vi "1.vi"   [LabVIEW 2015]
doc: "This VI is called when autonomous begins, and will automatically be terminated when autonomous ends. You can carry out timed or sensor driven robot movement independently without needing to return to the caller."
uses:
  <vilib>/Rock Robotics/WPI/Utilities/WPI_GetSetVariantRefNum.vi
  <vilib>/Rock Robotics/Network Tables/NT Read Number.vi
  <vilib>/Rock Robotics/WPI/RobotDrive/WPI_RobotDriveMecanumDrive_Cartesian.vi
  <vilib>/Rock Robotics/Network Tables/NT Write Numeric Array.vi
  Robot Global Data.vi
panel:
  # "Be sure to right-click and choose Data Operations>>Make Current Value default if you want to save the array values with the VI"
types:
  T1 = typedef "WPI_JoystickDevRef.ctl" = cluster{"Device":T2}
  T2 = typedef "WPI_JoystickDeviceEnum.ctl" = enum16{"USB 0", "USB 1", "USB 2", "USB 3", "USB 4", "USB 5"}
  T3 = typedef "WPI_RobotDriveDevRef.ctl" = cluster{"DevStatus":errorcluster, "Motors[]":T4[], "Square Inputs":bool, "Max Output":dbl}
  T4 = typedef "WPI_MotorControlDeviceRef.ctl" = cluster{"DeviceStatus":errorcluster, "Type":T5, "PWM":cluster{"PWM Channel":T6, "DeadBand":T7}, "CAN":cluster{"Device Number":u8, "Control Mode":T8, "Semaphore":T9, "Max Vout":dbl, "TalonSRX Control Mode":T10}, "Invert":bool}
  T5 = typedef "WPI_MotorControlType.ctl" = enum16{"PWM", "CAN", "CANTalonSRX"}
  T6 = typedef "FPGA_DIOPWMChannel.ctl" = enum8{"PWM 0", "PWM 1", "PWM 2", "PWM 3", "PWM 4", "PWM 5", "PWM 6", "PWM 7", "PWM 8", "PWM 9", "PWM MXP 0", "PWM MXP 1", "PWM MXP 2", "PWM MXP 3", "PWM MXP 4", "PWM MXP 5", "PWM MXP 6", "PWM MXP 7", "PWM MXP 8", "PWM MXP 9", "Invalid"}
  T7 = typedef "WPI_PWMDeadband.ctl" = cluster{"Name":string, "maxPositivePwm":i32, "minPositivePwm":i32, "centerPwm":i32, "maxNegativePwm":i32, "minNegativePwm":i32, "angularRange":u16}
  T8 = typedef "WPI_CANJaguar_ControlMode.ctl" = enum8{"Percent VBus", "Current", "Speed", "Position", "Voltage"}
  T9 = typedef "Semaphore RefNum" = refnum<k1>
  T10 = typedef "WPI_CANTalonSRX_APIControlMode.ctl" = enum8{"Percent VBus", "Speed", "Position", "Slave", "Unchanged / Invalid", "Voltage Compensation", "Current", "Motion Profile"}
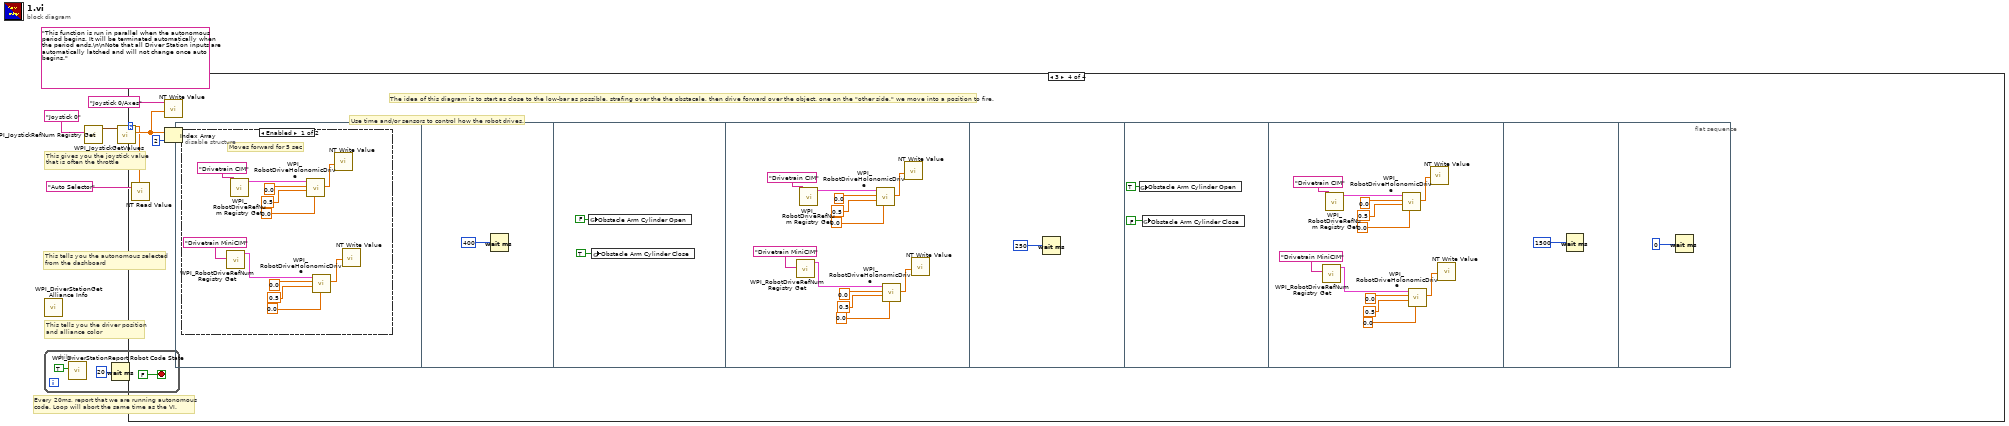
[diagram p0: block diagram]
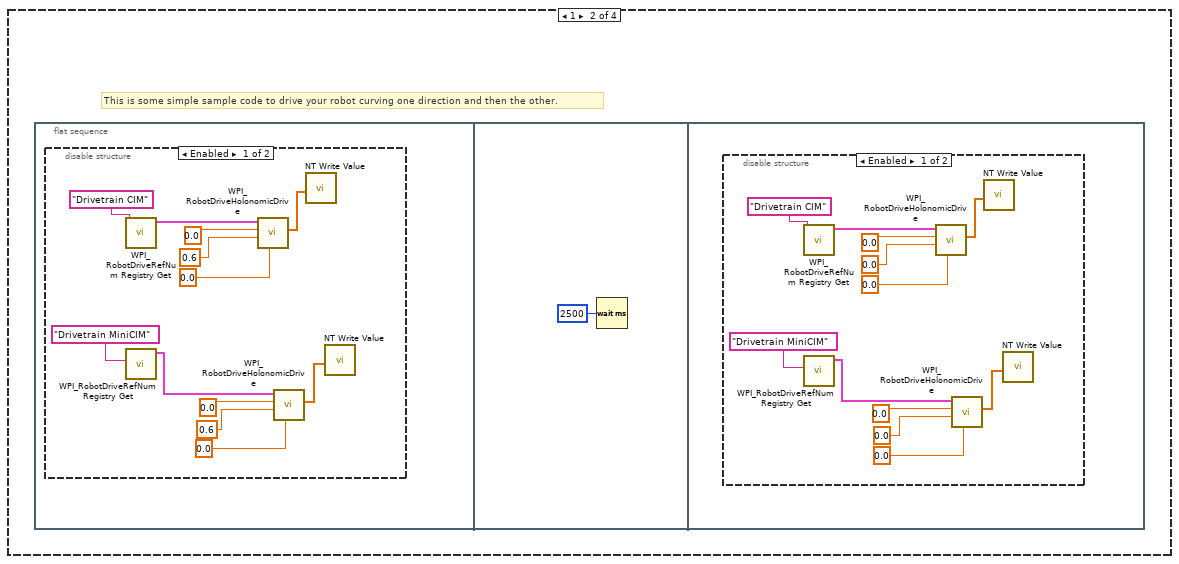
[diagram p3: hidden frame]
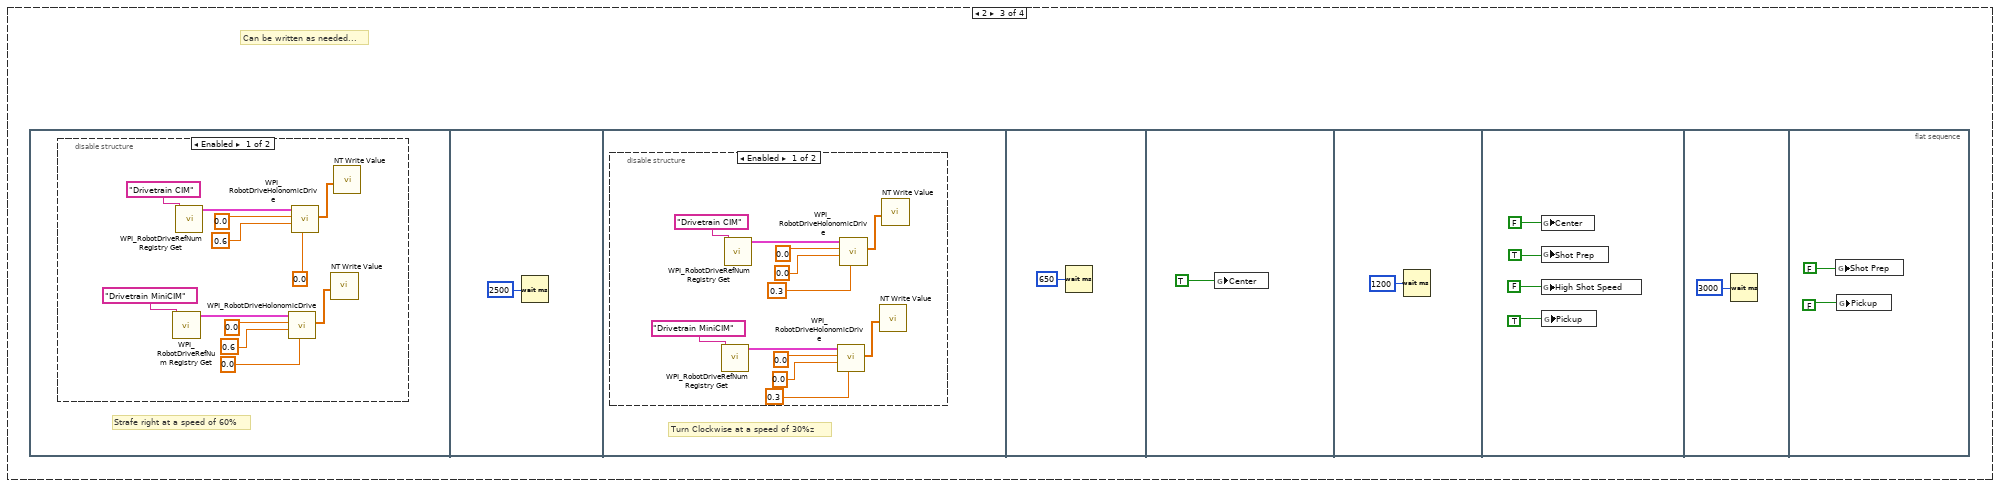
[diagram p6: hidden frame]
diagram:
  (unwired) "This function is run in parallel when the autonomous period begins. It will be terminated automatically when the period ends.\n\nNote that all Driver Station inputs are automatically latched and will not change once auto begins."
  # "This tells you the autonomous selected\nfrom the dashboard"
  # "Every 20ms, report that we are running autonomous\ncode. Loop will abort the same time as the VI."
  # "This gives you the joystick value\nthat is often the throttle"
  # "Use time and/or sensors to control how the robot drives."
  # "This tells you the driver position\nand alliance color"
  n1 = while {
    stop <- FALSE stop-if-true
    n2 = call <vilib>:"WPI_DriverStationReport Robot Code State.vi"("Autonomous"=TRUE) -> ()  [unwired: 10 in, 1 out]
    n3 = Wait (ms)(milliseconds to wait=u32 20) -> ()  [unwired: 1 out]
  }
  n4 = call <vilib>:"WPI_DriverStationGet Alliance Info.vi"() -> ()  [unwired: 12 out]
  n5 = call <vilib>:"WPI_JoystickRefNum Registry Get.vi"("refnum name"="Joystick 0") -> ("JoystickDevRef"=w6:T1)  [unwired: 1 in, 9 out]
  n6 = call <vilib>:"WPI_JoystickGetValues.vi"("JoystickDevRef"=w6) -> ("Axes"=w3:dbl[])  [unwired: 6 in, 4 out]
  n7 = call-poly <vilib>:"NT Read Value.vi"("Name"="Auto Selector") -> ("Numeric"=w1:dbl)  [unwired: 9 in, 1 out]
  n8 = case shown="3" w1 {
    frame 0, Default {
    }
    frame 1 {
      # "This is some simple sample code to drive your robot curving one direction and then the other."
      n9 = flat-sequence {
        frame #0 {
          n10 = disable-structure shown="Enabled" {
            frame Enabled {
              n11 = call <vilib>:"WPI_RobotDriveRefNum Registry Get.vi"("refnum name"="Drivetrain CIM") -> ("RobotDriveDevRef"=w18:T3)  [unwired: 1 in, 9 out]
              n12 = call <vilib>:"WPI_RobotDriveRefNum Registry Get.vi"("refnum name"="Drivetrain MiniCIM") -> ("RobotDriveDevRef"=w12:T3)  [unwired: 1 in, 9 out]
              n13 = call-poly <vilib>:"WPI_RobotDriveHolonomicDrive.vi"("Rotation"=0.0, "Y"=0.6 ("X axis value"), "X"=0.0 ("X axis value"), "RobotDriveDevRef"=w18) -> ("Motor Values"=w19:dbl[])  [unwired: 5 in, 2 out]
              n14 = call-poly <vilib>:"WPI_RobotDriveHolonomicDrive.vi"("Rotation"=0.0, "Y"=0.6 ("X axis value"), "X"=0.0 ("X axis value"), "RobotDriveDevRef"=w12) -> ("Motor Values"=w14:dbl[])  [unwired: 5 in, 2 out]
              n15 = call-poly <vilib>:"NT Write Value.vi"("Numeric Array"=w19) -> ()  [unwired: 10 in, 1 out]
              n16 = call-poly <vilib>:"NT Write Value.vi"("Numeric Array"=w14) -> ()  [unwired: 10 in, 1 out]
            }
            frame Disabled {
            }
          }
        }
        frame #1 {
          n17 = Wait (ms)(milliseconds to wait=u32 2500) -> ()  [unwired: 1 out]
        }
        frame #2 {
          n18 = disable-structure shown="Enabled" {
            frame Enabled {
              n19 = call <vilib>:"WPI_RobotDriveRefNum Registry Get.vi"("refnum name"="Drivetrain CIM") -> ("RobotDriveDevRef"=w31:T3)  [unwired: 1 in, 9 out]
              n20 = call <vilib>:"WPI_RobotDriveRefNum Registry Get.vi"("refnum name"="Drivetrain MiniCIM") -> ("RobotDriveDevRef"=w25:T3)  [unwired: 1 in, 9 out]
              n21 = call-poly <vilib>:"WPI_RobotDriveHolonomicDrive.vi"("Rotation"=0.0, "Y"=0.0 ("X axis value"), "X"=0.0 ("X axis value"), "RobotDriveDevRef"=w31) -> ("Motor Values"=w32:dbl[])  [unwired: 5 in, 2 out]
              n22 = call-poly <vilib>:"WPI_RobotDriveHolonomicDrive.vi"("Rotation"=0.0, "Y"=0.0 ("X axis value"), "X"=0.0 ("X axis value"), "RobotDriveDevRef"=w25) -> ("Motor Values"=w27:dbl[])  [unwired: 5 in, 2 out]
              n23 = call-poly <vilib>:"NT Write Value.vi"("Numeric Array"=w32) -> ()  [unwired: 10 in, 1 out]
              n24 = call-poly <vilib>:"NT Write Value.vi"("Numeric Array"=w27) -> ()  [unwired: 10 in, 1 out]
            }
            frame Disabled {
            }
          }
        }
      }
    }
    frame 2 {
      # "Can be written as needed..."
      n25 = flat-sequence {
        frame #0 {
          # "Strafe right at a speed of 60%"
          n26 = disable-structure shown="Enabled" {
            frame Enabled {
              n27 = call <vilib>:"WPI_RobotDriveRefNum Registry Get.vi"("refnum name"="Drivetrain MiniCIM") -> ("RobotDriveDevRef"=w37:T3)  [unwired: 1 in, 9 out]
              n28 = call <vilib>:"WPI_RobotDriveRefNum Registry Get.vi"("refnum name"="Drivetrain CIM") -> ("RobotDriveDevRef"=w43:T3)  [unwired: 1 in, 9 out]
              n29 = call-poly <vilib>:"WPI_RobotDriveHolonomicDrive.vi"("Rotation"=0.0, "Y"=0.6 ("X axis value"), "X"=0.0 ("X axis value"), "RobotDriveDevRef"=w37) -> ("Motor Values"=w38:dbl[])  [unwired: 5 in, 2 out]
              n30 = call-poly <vilib>:"WPI_RobotDriveHolonomicDrive.vi"("Rotation"=0.0, "Y"=0.6 ("X axis value"), "X"=0.0 ("X axis value"), "RobotDriveDevRef"=w43) -> ("Motor Values"=w44:dbl[])  [unwired: 5 in, 2 out]
              n31 = call-poly <vilib>:"NT Write Value.vi"("Numeric Array"=w38) -> ()  [unwired: 10 in, 1 out]
              n32 = call-poly <vilib>:"NT Write Value.vi"("Numeric Array"=w44) -> ()  [unwired: 10 in, 1 out]
            }
            frame Disabled {
            }
          }
        }
        frame #1 {
          n33 = Wait (ms)(milliseconds to wait=u32 2500) -> ()  [unwired: 1 out]
        }
        frame #2 {
          # "Turn Clockwise at a speed of 30%z"
          n34 = disable-structure shown="Enabled" {
            frame Enabled {
              n35 = call <vilib>:"WPI_RobotDriveRefNum Registry Get.vi"("refnum name"="Drivetrain MiniCIM") -> ("RobotDriveDevRef"=w50:T3)  [unwired: 1 in, 9 out]
              n36 = call <vilib>:"WPI_RobotDriveRefNum Registry Get.vi"("refnum name"="Drivetrain CIM") -> ("RobotDriveDevRef"=w56:T3)  [unwired: 1 in, 9 out]
              n37 = call-poly <vilib>:"WPI_RobotDriveHolonomicDrive.vi"("Rotation"=0.3, "Y"=0.0 ("X axis value"), "X"=0.0 ("X axis value"), "RobotDriveDevRef"=w50) -> ("Motor Values"=w51:dbl[])  [unwired: 5 in, 2 out]
              n38 = call-poly <vilib>:"WPI_RobotDriveHolonomicDrive.vi"("Rotation"=0.3, "Y"=0.0 ("X axis value"), "X"=0.0 ("X axis value"), "RobotDriveDevRef"=w56) -> ("Motor Values"=w57:dbl[])  [unwired: 5 in, 2 out]
              n39 = call-poly <vilib>:"NT Write Value.vi"("Numeric Array"=w51) -> ()  [unwired: 10 in, 1 out]
              n40 = call-poly <vilib>:"NT Write Value.vi"("Numeric Array"=w57) -> ()  [unwired: 10 in, 1 out]
            }
            frame Disabled {
            }
          }
        }
        frame #3 {
          n41 = Wait (ms)(milliseconds to wait=u32 650) -> ()  [unwired: 1 out]
        }
        frame #4 {
          n42 = global write "Robot Global Data.vi" "Center"(TRUE) -> ()
        }
        frame #5 {
          n43 = Wait (ms)(milliseconds to wait=u32 1200) -> ()  [unwired: 1 out]
        }
        frame #6 {
          n44 = global write "Robot Global Data.vi" "Center"(FALSE) -> ()
          n45 = global write "Robot Global Data.vi" "Shot Prep"(TRUE) -> ()
          n46 = global write "Robot Global Data.vi" "High Shot Speed"(FALSE) -> ()
          n47 = global write "Robot Global Data.vi" "Pickup"(TRUE) -> ()
        }
        frame #7 {
          n48 = Wait (ms)(milliseconds to wait=u32 3000) -> ()  [unwired: 1 out]
        }
        frame #8 {
          n49 = global write "Robot Global Data.vi" "Shot Prep"(FALSE) -> ()
          n50 = global write "Robot Global Data.vi" "Pickup"(FALSE) -> ()
        }
      }
    }
    frame 3 {
      # "The idea of this diagram is to start as close to the low-bar as possible, strafing over the the obstacale, then drive forward over the object. one on the \"other side,\" we move into a position to fire."
      n51 = flat-sequence {
        frame #0 {
          n52 = disable-structure shown="Enabled" {
            frame Enabled {
              # "Moves forward for 5 sec"
              n53 = call <vilib>:"WPI_RobotDriveRefNum Registry Get.vi"("refnum name"="Drivetrain MiniCIM") -> ("RobotDriveDevRef"=w72:T3)  [unwired: 1 in, 9 out]
              n54 = call <vilib>:"WPI_RobotDriveRefNum Registry Get.vi"("refnum name"="Drivetrain CIM") -> ("RobotDriveDevRef"=w78:T3)  [unwired: 1 in, 9 out]
              n55 = call-poly <vilib>:"WPI_RobotDriveHolonomicDrive.vi"("Rotation"=0.0, "Y"=0.5 ("X axis value"), "X"=0.0 ("X axis value"), "RobotDriveDevRef"=w78) -> ("Motor Values"=w79:dbl[])  [unwired: 5 in, 2 out]
              n56 = call-poly <vilib>:"WPI_RobotDriveHolonomicDrive.vi"("Rotation"=0.0, "Y"=0.5 ("X axis value"), "X"=0.0 ("X axis value"), "RobotDriveDevRef"=w72) -> ("Motor Values"=w74:dbl[])  [unwired: 5 in, 2 out]
              n57 = call-poly <vilib>:"NT Write Value.vi"("Numeric Array"=w79) -> ()  [unwired: 10 in, 1 out]
              n58 = call-poly <vilib>:"NT Write Value.vi"("Numeric Array"=w74) -> ()  [unwired: 10 in, 1 out]
            }
            frame Disabled {
            }
          }
        }
        frame #1 {
          n59 = Wait (ms)(milliseconds to wait=u32 400) -> ()  [unwired: 1 out]
        }
        frame #2 {
          n60 = global write "Robot Global Data.vi" "Obstacle Arm Cylinder Open"(FALSE) -> ()
          n61 = global write "Robot Global Data.vi" "Obstacle Arm Cylinder Close"(TRUE) -> ()
        }
        frame #3 {
          n62 = call <vilib>:"WPI_RobotDriveRefNum Registry Get.vi"("refnum name"="Drivetrain MiniCIM") -> ("RobotDriveDevRef"=w87:T3)  [unwired: 1 in, 9 out]
          n63 = call <vilib>:"WPI_RobotDriveRefNum Registry Get.vi"("refnum name"="Drivetrain CIM") -> ("RobotDriveDevRef"=w93:T3)  [unwired: 1 in, 9 out]
          n64 = call-poly <vilib>:"WPI_RobotDriveHolonomicDrive.vi"("Rotation"=0.0, "Y"=0.5 ("X axis value"), "X"=0.0 ("X axis value"), "RobotDriveDevRef"=w93) -> ("Motor Values"=w94:dbl[])  [unwired: 5 in, 2 out]
          n65 = call-poly <vilib>:"WPI_RobotDriveHolonomicDrive.vi"("Rotation"=0.0, "Y"=0.5 ("X axis value"), "X"=0.0 ("X axis value"), "RobotDriveDevRef"=w87) -> ("Motor Values"=w89:dbl[])  [unwired: 5 in, 2 out]
          n66 = call-poly <vilib>:"NT Write Value.vi"("Numeric Array"=w94) -> ()  [unwired: 10 in, 1 out]
          n67 = call-poly <vilib>:"NT Write Value.vi"("Numeric Array"=w89) -> ()  [unwired: 10 in, 1 out]
        }
        frame #4 {
          n68 = Wait (ms)(milliseconds to wait=u32 250) -> ()  [unwired: 1 out]
        }
        frame #5 {
          n69 = global write "Robot Global Data.vi" "Obstacle Arm Cylinder Open"(TRUE) -> ()
          n70 = global write "Robot Global Data.vi" "Obstacle Arm Cylinder Close"(FALSE) -> ()
        }
        frame #6 {
          n71 = call <vilib>:"WPI_RobotDriveRefNum Registry Get.vi"("refnum name"="Drivetrain MiniCIM") -> ("RobotDriveDevRef"=w102:T3)  [unwired: 1 in, 9 out]
          n72 = call <vilib>:"WPI_RobotDriveRefNum Registry Get.vi"("refnum name"="Drivetrain CIM") -> ("RobotDriveDevRef"=w108:T3)  [unwired: 1 in, 9 out]
          n73 = call-poly <vilib>:"WPI_RobotDriveHolonomicDrive.vi"("Rotation"=0.0, "Y"=0.5 ("X axis value"), "X"=0.0 ("X axis value"), "RobotDriveDevRef"=w108) -> ("Motor Values"=w109:dbl[])  [unwired: 5 in, 2 out]
          n74 = call-poly <vilib>:"WPI_RobotDriveHolonomicDrive.vi"("Rotation"=0.0, "Y"=0.5 ("X axis value"), "X"=0.0 ("X axis value"), "RobotDriveDevRef"=w102) -> ("Motor Values"=w104:dbl[])  [unwired: 5 in, 2 out]
          n75 = call-poly <vilib>:"NT Write Value.vi"("Numeric Array"=w109) -> ()  [unwired: 10 in, 1 out]
          n76 = call-poly <vilib>:"NT Write Value.vi"("Numeric Array"=w104) -> ()  [unwired: 10 in, 1 out]
        }
        frame #7 {
          n77 = Wait (ms)(milliseconds to wait=u32 1500) -> ()  [unwired: 1 out]
        }
        frame #8 {
          n78 = Wait (ms)(milliseconds to wait=u32 0) -> ()  [unwired: 1 out]
        }
      }
    }
  }
  n79 = call-poly <vilib>:"NT Write Value.vi"("Numeric Array"=w3, "Name"="Joystick 0/Axes") -> ()  [unwired: 9 in, 1 out]
  n80 = Index Array(array=w3, index=2) -> ()  [unwired: 1 out]
